vi "Main_Daily_path.vi"(10 "nothing":bool) -> (2 "Directory path(STR)":string, 3 "Directory path":path)   [LabVIEW 2017]
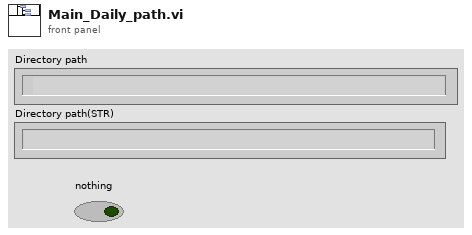
[diagram p1: front panel]
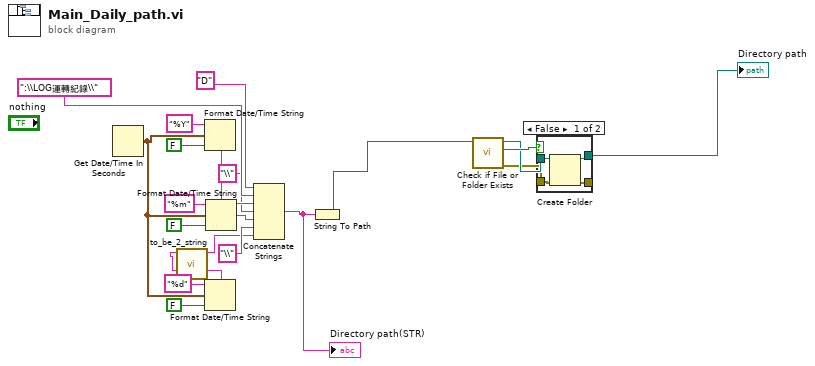
[diagram p0: block diagram]
diagram:
  n1 = Get Date/Time In Seconds() -> (seconds since 1Jan1904=w21:timestamp)
  n2 = Format Date/Time String(time format string (%c)="%Y", seconds (now)=w21, UTC format=FALSE) -> (date/time string=w15:string)
  n3 = Format Date/Time String(time format string (%c)="%d", seconds (now)=w21, UTC format=FALSE) -> (date/time string=w7:string)
  n4 = call "to_be_2_string.vi"("string 2"=w7) -> ("substring 2"=w6:string)  [unwired: 10 in]
  n5 = Format Date/Time String(time format string (%c)="%m", seconds (now)=w21, UTC format=FALSE) -> (date/time string=w11:string)
  n6 = Concatenate Strings("D" ("磁碟位置"), ":\\LOG運轉紀錄\\", w15, "\\", w11, "\\", w6) -> (w19:string)
  "Directory path(STR)" <- w19
  n7 = String To Path(string=w19) -> (path=w2:path)
  n8 = call <vilib>:"Check if File or Folder Exists.vi"("path"=w2) -> ("error out"=w3:errorcluster, "file or folder exists?"=w5:bool, "dup path"=w4:path)  [unwired: 8 in]
  n9 = case shown="False" w5 {
    tunnel: w4 -> [w25 w26]
    tunnel: [w24 w27] -> _
    tunnel: w3 -> [w23 w27]
    tunnel: [w22 w26] -> w1
    frame False {
      n10 = Create Folder(path (use dialog)=w25, error in=w23) -> (created path=w22:path, error out=w24:errorcluster)  [unwired: 1 in, 1 out]
    }
    frame True {
    }
  }
  "Directory path" <- w1
